vi "Wire All Terminals_core.vi"(8 "error in (no error)":errorcluster, 9 "User string":string, 10 "Create constants?":bool, 11 "SelList[]":refnum<vi>[](array[refnum])) -> (0 "error out":errorcluster, 3 "changes made?":bool)   [LabVIEW 2020]
doc: "Creates controls and indicators for all unwired inputs and outputs of the selected block diagram object(s). If 'shift' is also pressed, creates constants for all unwired inputs of the selected block diagram object(s).\n\nDefault Shortcut - [D]"
uses:
  <resource>/plugins/PopupMenus/edit time panel and diagram/zzRemove (no error).llb/zzRemove (no error).ctl
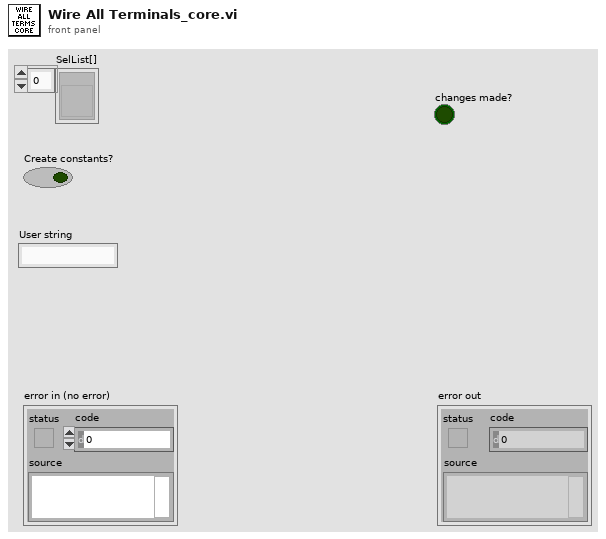
[diagram p1: front panel]
types:
  T1 = typedef "zzRemove (no error).ctl" = cluster{"Terminals":refnum<vi>[]}
  T2 = enum16{"Invalid Wire Rule", "Required", "Recommended", "Optional", "Dynamic Dispatch"}[]
  T3 = typedef "NI_Data Type.lvlib/Data Type.ctl" = enum8{"Invalid Type", "Void", "I8", "I16", "I32", "I64", "U8", "U16", "U32", "U64", "Single Float", "Double Float", "Extended Float", "Single Complex", "Double Complex", "Extended Complex", "Enum U8", "Enum U16", "Enum U32", "Enum U64", "Single Float With Unit", "Double Float With Unit", "Extended Float With Unit", "Single Complex with Unit", "Double Complex with Unit", "Extended Complex with Unit", "Boolean", "String", "Path", "Picture", "Tag", "Array", "Cluster", "Variant", "LV Variant", "Waveform", "Timestamp", "Digital Waveform", "Digital Data", "ExpressData", "Refnum", "External Data", "VI", "Poly VI", "LabVIEW Class Instance", "Fixed Point", "Set Collection", "Map Collection"}
  T4 = enum16{"Invalid Wire Rule", "Required", "Recommended", "Optional"}
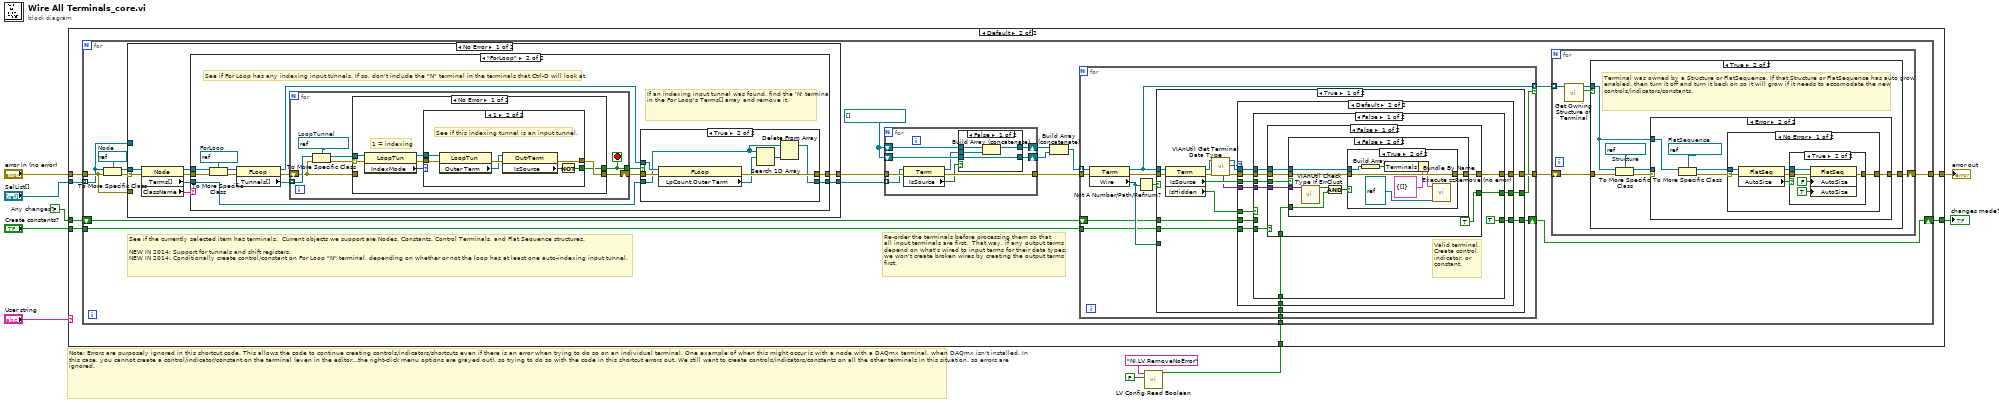
[diagram p0: block diagram]
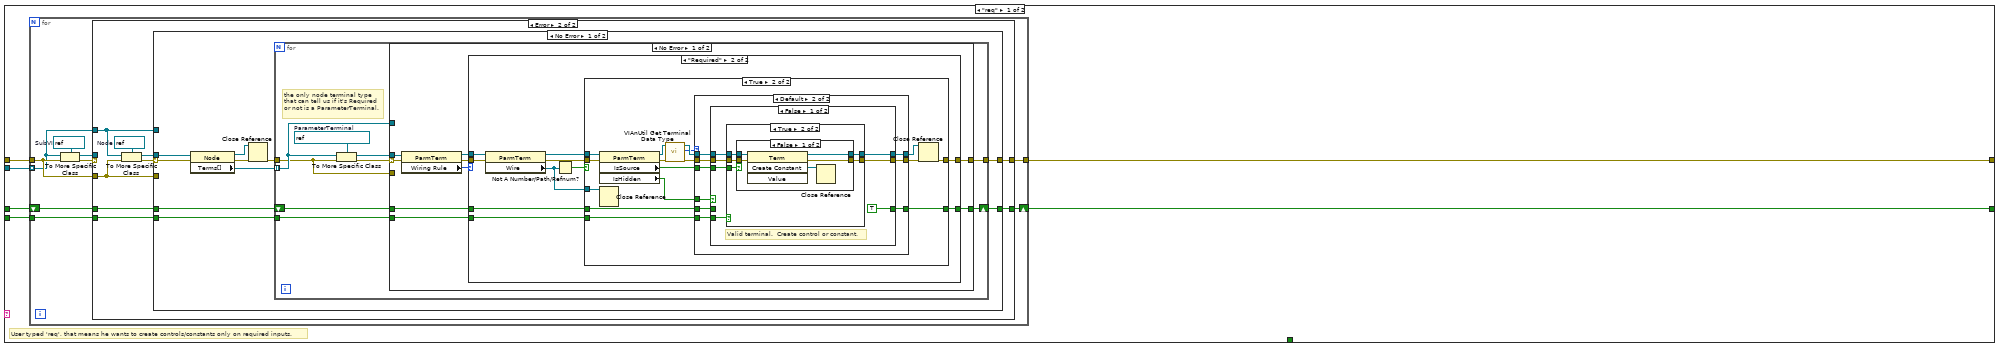
[diagram p2: hidden frame]
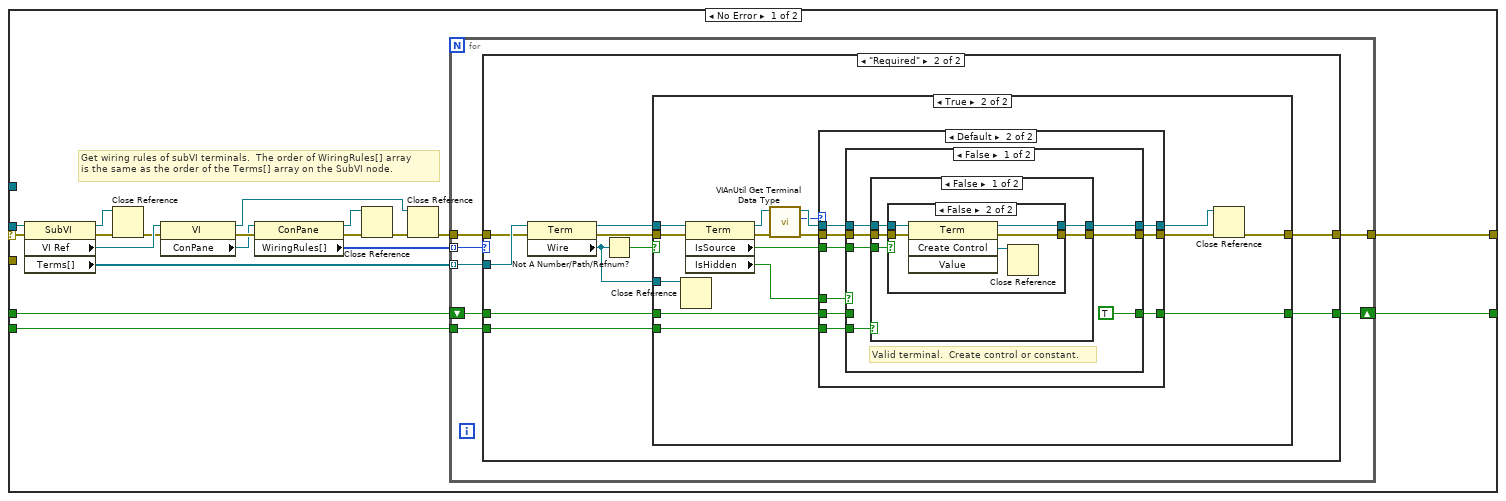
[diagram p3: hidden frame]
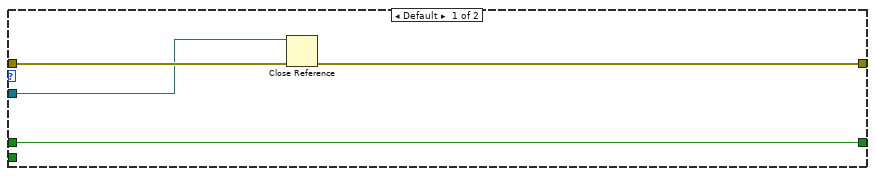
[diagram p4: hidden frame]
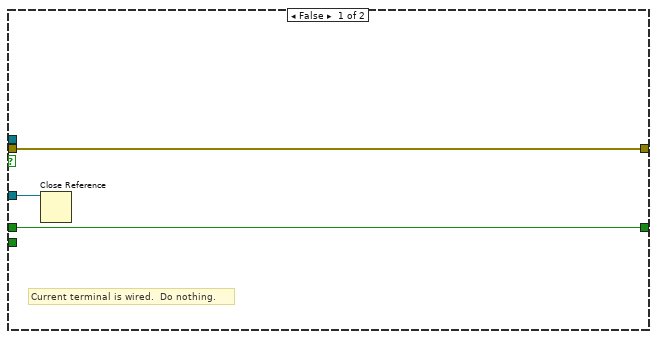
[diagram p5: hidden frame]
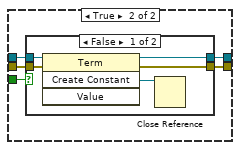
[diagram p8: hidden frame]
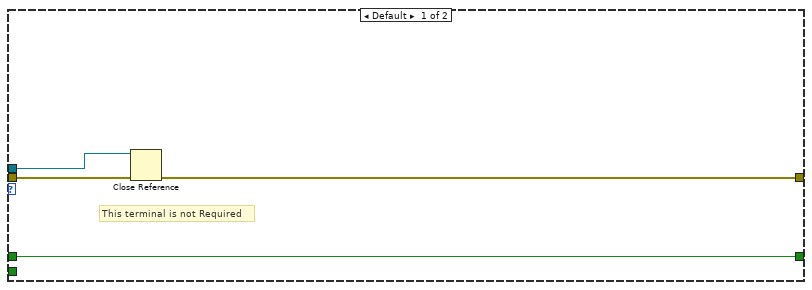
[diagram p11: hidden frame]
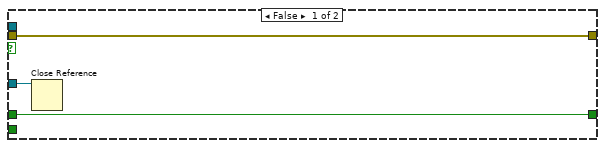
[diagram p12: hidden frame]
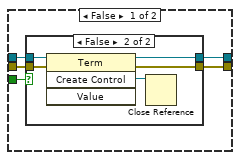
[diagram p14: hidden frame]
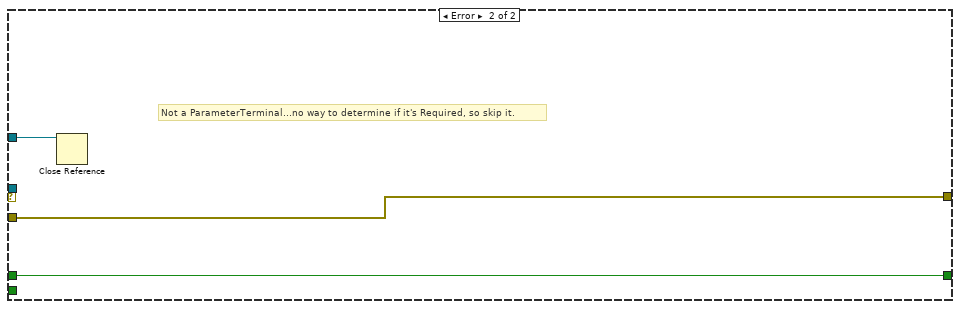
[diagram p18: hidden frame]
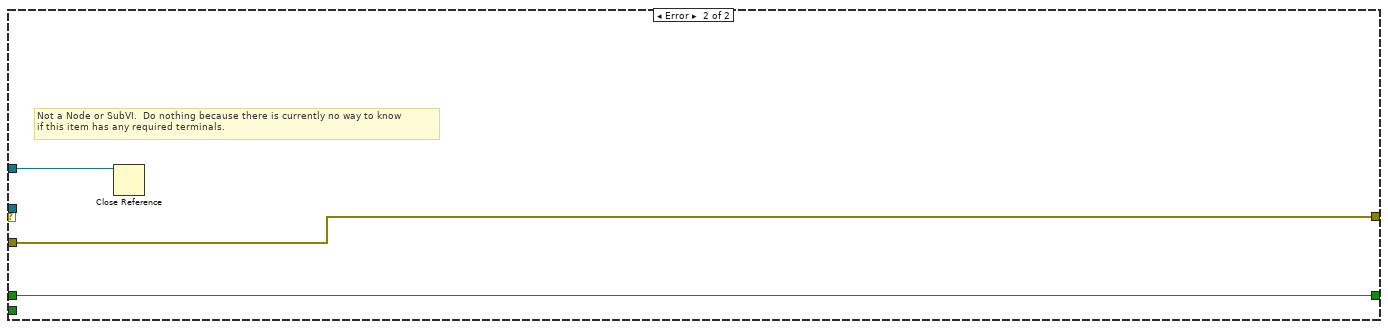
[diagram p19: hidden frame]
diagram:
  w10 = FALSE  # Any changes?
  # "Note: Errors are purposely ignored in this shortcut code. This allows the code to continue creating controls/indicators/shortcuts even if there is an error when trying to do so on an individual terminal. One example of when this might occur is with a node with a DAQmx terminal, when DAQmx isn't installed. In this case, you cannot create a control/indicator/constant on the terminal (even in the editor...the right-click menu options are grayed out), so trying to do so with the code in this shortcut errors out. We still want to create controls/indicators/constants on all the other terminals in this situation, so errors are ignored."
  n1 = call <resource>:"LV Config Read Boolean.vi"("default value"=FALSE, "key"="NI.LV.RemoveNoError") -> ("value"=w1:bool)  [unwired: 3 in, 2 out]
  n2 = case shown="Default" "User string" {
    tunnel: "Create constants?" -> [w11 w259]
    tunnel: w10 -> [w16 w258]
    tunnel: [w15 w257] -> w7
    tunnel: [w12 w256] -> w8
    tunnel: "SelList[]" -> [w14 w255]
    tunnel: "error in (no error)" -> [w13 w254]
    tunnel: w1 -> [_ w253]
    frame "req" {
      # "User typed 'req', that means he wants to create controls/constants only on required inputs."
      n3 = for {
        shift-right: [w20] -> w15
        shift-left: w16 -> [w22]
        tunnel: w14 -> [w17] mode=indexing
        tunnel: w11 -> [w19]
        tunnel: w13 -> [w18]
        tunnel: [w21] -> w12
        w25 = refnum<vi> refnum  # SubVI
        n4 = To More Specific Class(target class=w25, reference=w17, error in=w18) -> (specific class reference=w23:refnum<vi>, error out=w24:errorcluster)
        n5 = case shown="Error" w24 {
          selector: w24 -> [w43 _]
          tunnel: w23 -> [w44 _]
          tunnel: w22 -> [w30 w132]
          tunnel: [w33 w134] -> w21
          tunnel: [w29 w133] -> w20
          tunnel: w19 -> [w28 w131]
          tunnel: w18 -> [_ w137]
          tunnel: w17 -> [_ w135]
          frame No Error {
            # "Get wiring rules of subVI terminals.  The order of WiringRules[] array\nis the same as the order of the Terms[] array on the SubVI node."
            n6 = property class="SubVI"(reference=w44, error in=w43) -> (reference out=w26:refnum<vi>, error out=w42:errorcluster, "VI Ref"=w41:refnum<vi>, "Terms[]"=w31:refnum<vi>[])
            n7 = Close Reference(reference=w26, error in (no error)=w42) -> (error out=w27:errorcluster)
            n8 = property class="VI"(reference=w41, error in=w27) -> (reference out=w35:refnum<vi>, error out=w40:errorcluster, "ConPane"=w39:refnum<vi>)
            n9 = property class="ConPane"(reference=w39, error in=w40) -> (reference out=w37:refnum<vi>, error out=w38:errorcluster, "WiringRules[]"=w32:T2)
            n10 = Close Reference(reference=w37, error in (no error)=w38) -> (error out=w36:errorcluster)
            n11 = Close Reference(reference=w35, error in (no error)=w36) -> (error out=w34:errorcluster)
            n12 = for {
              tunnel: w32 -> [w50] mode=indexing
              tunnel: w31 -> [w49] mode=indexing
              shift-right: [w46] -> w29
              shift-left: w30 -> [w47]
              tunnel: w28 -> [w45]
              tunnel: w34 -> [w51]
              tunnel: [w48] -> w33
              n13 = case shown="\"Required\"" w50 {
                tunnel: w51 -> [w55 w57]
                tunnel: w49 -> [w52 w61]
                tunnel: [w54 w62] -> w48
                tunnel: w47 -> [w53 w65]
                tunnel: [w53 w63] -> w46
                tunnel: w45 -> [_ w64]
                frame Default {
                  n14 = Close Reference(reference=w52, error in (no error)=w55) -> (error out=w54:errorcluster)
                }
                frame "Required" {
                  n15 = property class="Term"(reference=w61, error in=w57) -> (reference out=w60:refnum<vi>, error out=w56:errorcluster, "Wire"=w58:refnum<vi>)
                  n16 = Not A Number/Path/Refnum?(number/path/refnum=w58) -> (NaN/Path/Refnum?=w59:bool)
                  n17 = case shown="True" w59 {
                    tunnel: w65 -> [w66 w80]
                    tunnel: w64 -> [_ w79]
                    tunnel: [w66 w78] -> w63
                    tunnel: [w67 w77] -> w62
                    tunnel: w56 -> [w67 w76]
                    tunnel: w60 -> [_ w70]
                    tunnel: w58 -> [w68 w69]
                    frame False {
                      # "Current terminal is wired.  Do nothing."
                      n18 = Close Reference(reference=w68) -> ()  [unwired: 1 in, 1 out]
                    }
                    frame True {
                      n19 = Close Reference(reference=w69) -> ()  [unwired: 1 in, 1 out]
                      n20 = property class="Term"(reference=w70, error in=w76) -> (reference out=w73:refnum<vi>, error out=w75:errorcluster, "IsSource"=w84:bool, "IsHidden"=w81:bool)
                      n21 = call <vilib>:"VIAnUtil Get Terminal Data Type.vi"("error in (no error)"=w75, "Terminal in"=w73) -> ("error out"=w74:errorcluster, "Data Type"=w71:T3, "Terminal out"=w72:refnum<vi>)  [unwired: 6 in, 1 out]
                      n22 = case shown="Default" w71 {
                        tunnel: [w87 w96] -> w78
                        tunnel: w84 -> [_ w95]
                        tunnel: w72 -> [w85 w94]
                        tunnel: [w86 w93] -> w83
                        tunnel: [w85 w92] -> w82
                        tunnel: w74 -> [w86 w91]
                        tunnel: w80 -> [w87 w88]
                        tunnel: w79 -> [_ w90]
                        tunnel: w81 -> [_ w89]
                        frame "Invalid Type", "Void" {
                          # "Current terminal is void (like an empty terminal on\na subVI).  Do nothing."
                        }
                        frame Default {
                          n23 = case shown="False" w89 {
                            tunnel: [TRUE w128] -> w96
                            tunnel: w95 -> [w102 _]
                            tunnel: w94 -> [w101 w129]
                            tunnel: [w100 w130] -> w93
                            tunnel: [w99 w129] -> w92
                            tunnel: w91 -> [w98 w130]
                            tunnel: w90 -> [w97 _]
                            tunnel: w88 -> [_ w128]
                            frame False {
                              # "Valid terminal.  Create control or constant."
                              n24 = case shown="False" w97 {
                                tunnel: w102 -> [w108 w120]
                                tunnel: w101 -> [w107 w119]
                                tunnel: [w106 w118] -> w100
                                tunnel: [w105 w117] -> w99
                                tunnel: w98 -> [w104 w116]
                                frame False {
                                n25 = case shown="False" w108 {
                                tunnel: w104 -> [w109 w115]
                                tunnel: w107 -> [w110 w113]
                                tunnel: [w109 w114] -> w106
                                tunnel: [w110 w112] -> w105
                                frame True {
                                }
                                frame False {
                                n26 = invoke class="Term" method="Create Control"(reference=w113, error in=w115) -> (reference out=w112:refnum<vi>, error out=w114:errorcluster, "Create Control"=w111:refnum<vi>)  [unwired: 2 in, 1 out]
                                n27 = Close Reference(reference=w111) -> ()  [unwired: 1 in, 1 out]
                                }
                                }
                                }
                                frame True {
                                n28 = case shown="False" w120 {
                                tunnel: w116 -> [w125 w127]
                                tunnel: w119 -> [w123 w126]
                                tunnel: [w124 w127] -> w118
                                tunnel: [w122 w126] -> w117
                                frame False {
                                n29 = invoke class="Term" method="Create Constant"(reference=w123, error in=w125) -> (reference out=w122:refnum<vi>, error out=w124:errorcluster, "Create Constant"=w121:refnum<vi>)  [unwired: 2 in, 1 out]
                                n30 = Close Reference(reference=w121) -> ()  [unwired: 1 in, 1 out]
                                }
                                frame True {
                                }
                                }
                                }
                              }
                            }
                            frame True {
                              # "Do not attempt to create inputs/outputs\non hidden terminals (like Dynamic Event terms\non an Event Structure that aren't showing)"
                            }
                          }
                        }
                      }
                      n31 = Close Reference(reference=w82, error in (no error)=w83) -> (error out=w77:errorcluster)
                    }
                  }
                }
              }
            }
          }
          frame Error {
            w139 = refnum<vi> refnum  # Node
            n32 = To More Specific Class(target class=w139, reference=w135, error in=w137) -> (specific class reference=w136:refnum<vi>, error out=w138:errorcluster)
            n33 = case shown="No Error" w138 {
              selector: w138 -> [w149 _]
              tunnel: w137 -> [_ w251]
              tunnel: w136 -> [w148 _]
              tunnel: w135 -> [_ w252]
              tunnel: [w141 w251] -> w134
              tunnel: [w142 w250] -> w133
              tunnel: w132 -> [w143 w250]
              tunnel: w131 -> [w140 _]
              frame No Error {
                n34 = property class="Node"(reference=w148, error in=w149) -> (reference out=w146:refnum<vi>, error out=w147:errorcluster, "Terms[]"=w144:refnum<vi>[])
                n35 = Close Reference(reference=w146, error in (no error)=w147) -> (error out=w145:errorcluster)
                n36 = for {
                  tunnel: w144 -> [w153] mode=indexing
                  shift-right: [w154] -> w142
                  shift-left: w143 -> [w155]
                  tunnel: w140 -> [w150]
                  tunnel: w145 -> [w152]
                  tunnel: [w151] -> w141
                  w158 = refnum<vi> refnum  # ParameterTerminal
                  # "the only node terminal type\nthat can tell us if it's Required\nor not is a ParameterTerminal."
                  n37 = To More Specific Class(target class=w158, reference=w153, error in=w152) -> (specific class reference=w156:refnum<vi>, error out=w157:errorcluster)
                  n38 = case shown="No Error" w157 {
                    selector: w157 -> [w167 _]
                    tunnel: w156 -> [w166 _]
                    tunnel: w155 -> [w165 w249]
                    tunnel: [w160 w249] -> w154
                    tunnel: w153 -> [_ w248]
                    tunnel: w152 -> [_ w247]
                    tunnel: [w161 w247] -> w151
                    tunnel: w150 -> [w159 _]
                    frame No Error {
                      n39 = property class="ParmTerm"(reference=w166, error in=w167) -> (reference out=w162:refnum<vi>, error out=w163:errorcluster, "Wiring Rule"=w164:T4)
                      n40 = case shown="\"Required\"" w164 {
                        tunnel: w165 -> [w168 w181]
                        tunnel: w163 -> [w171 w175]
                        tunnel: w162 -> [w170 w177]
                        tunnel: [w169 w179] -> w161
                        tunnel: [w168 w180] -> w160
                        tunnel: w159 -> [_ w178]
                        frame Default {
                          # "This terminal is not Required"
                          n41 = Close Reference(reference=w170, error in (no error)=w171) -> (error out=w169:errorcluster)
                        }
                        frame "Required" {
                          n42 = property class="ParmTerm"(reference=w177, error in=w175) -> (reference out=w176:refnum<vi>, error out=w174:errorcluster, "Wire"=w172:refnum<vi>)
                          n43 = Not A Number/Path/Refnum?(number/path/refnum=w172) -> (NaN/Path/Refnum?=w173:bool)
                          n44 = case shown="True" w173 {
                            tunnel: w176 -> [_ w196]
                            tunnel: w181 -> [w184 w195]
                            tunnel: [w184 w194] -> w180
                            tunnel: [w183 w193] -> w179
                            tunnel: w178 -> [_ w192]
                            tunnel: w174 -> [w183 w191]
                            tunnel: w172 -> [w182 w185]
                            frame False {
                              n45 = Close Reference(reference=w182) -> ()  [unwired: 1 in, 1 out]
                            }
                            frame True {
                              n46 = property class="ParmTerm"(reference=w196, error in=w191) -> (reference out=w189:refnum<vi>, error out=w190:errorcluster, "IsSource"=w200:bool, "IsHidden"=w197:bool)
                              n47 = Close Reference(reference=w185) -> ()  [unwired: 1 in, 1 out]
                              n48 = call <vilib>:"VIAnUtil Get Terminal Data Type.vi"("error in (no error)"=w190, "Terminal in"=w189) -> ("error out"=w187:errorcluster, "Data Type"=w186:T3, "Terminal out"=w188:refnum<vi>)  [unwired: 6 in, 1 out]
                              n49 = case shown="Default" w186 {
                                tunnel: [w203 w212] -> w194
                                tunnel: w200 -> [_ w211]
                                tunnel: w188 -> [w201 w210]
                                tunnel: [w202 w209] -> w199
                                tunnel: [w201 w208] -> w198
                                tunnel: w187 -> [w202 w207]
                                tunnel: w195 -> [w203 w204]
                                tunnel: w192 -> [_ w206]
                                tunnel: w197 -> [_ w205]
                                frame "Invalid Type", "Void" {
                                # "Current terminal is void (like an empty terminal on\na subVI).  Do nothing."
                                }
                                frame Default {
                                n50 = case shown="False" w205 {
                                tunnel: [TRUE w244] -> w212
                                tunnel: w211 -> [w218 _]
                                tunnel: w210 -> [w217 w245]
                                tunnel: [w216 w246] -> w209
                                tunnel: [w215 w245] -> w208
                                tunnel: w207 -> [w214 w246]
                                tunnel: w206 -> [w213 _]
                                tunnel: w204 -> [_ w244]
                                frame False {
                                # "Valid terminal.  Create control or constant."
                                n51 = case shown="True" w213 {
                                tunnel: w218 -> [w224 w236]
                                tunnel: w217 -> [w223 w235]
                                tunnel: [w222 w234] -> w216
                                tunnel: [w221 w233] -> w215
                                tunnel: w214 -> [w220 w232]
                                frame False {
                                n52 = case shown="False" w224 {
                                tunnel: w220 -> [w225 w231]
                                tunnel: w223 -> [w226 w229]
                                tunnel: [w225 w230] -> w222
                                tunnel: [w226 w228] -> w221
                                frame True {
                                }
                                frame False {
                                n53 = invoke class="Term" method="Create Control"(reference=w229, error in=w231) -> (reference out=w228:refnum<vi>, error out=w230:errorcluster, "Create Control"=w227:refnum<vi>)  [unwired: 2 in, 1 out]
                                n54 = Close Reference(reference=w227) -> ()  [unwired: 1 in, 1 out]
                                }
                                }
                                }
                                frame True {
                                n55 = case shown="False" w236 {
                                tunnel: w232 -> [w241 w243]
                                tunnel: w235 -> [w239 w242]
                                tunnel: [w240 w243] -> w234
                                tunnel: [w238 w242] -> w233
                                frame False {
                                n56 = invoke class="Term" method="Create Constant"(reference=w239, error in=w241) -> (reference out=w238:refnum<vi>, error out=w240:errorcluster, "Create Constant"=w237:refnum<vi>)  [unwired: 2 in, 1 out]
                                n57 = Close Reference(reference=w237) -> ()  [unwired: 1 in, 1 out]
                                }
                                frame True {
                                }
                                }
                                }
                                }
                                }
                                frame True {
                                # "Do not attempt to create inputs/outputs\non hidden terminals (like Dynamic Event terms\non an Event Structure that aren't showing)"
                                }
                                }
                                }
                              }
                              n58 = Close Reference(reference=w198, error in (no error)=w199) -> (error out=w193:errorcluster)
                            }
                          }
                        }
                      }
                    }
                    frame Error {
                      # "Not a ParameterTerminal...no way to determine if it's Required, so skip it."
                      n59 = Close Reference(reference=w248) -> ()  [unwired: 1 in, 1 out]
                    }
                  }
                }
              }
              frame Error {
                # "Not a Node or SubVI.  Do nothing because there is currently no way to know\nif this item has any required terminals."
                n60 = Close Reference(reference=w252) -> ()  [unwired: 1 in, 1 out]
              }
            }
          }
        }
      }
    }
    frame Default {
      n61 = for {
        tunnel: w255 -> [w272] mode=indexing
        shift-right: [w261] -> w257
        shift-left: w258 -> [w276]
        tunnel: w259 -> [w275]
        tunnel: w254 -> [w274]
        tunnel: [w263] -> w256
        tunnel: w253 -> [w260]
        w267 = refnum<vi>[] [] ("Terms[]")
        w278 = refnum<vi> refnum  # Node
        # "Re-order the terminals before processing them so that\nall input terminals are first.  That way, if any output terms\ndepend on what's wired to input terms for their data types,\nwe won't create broken wires by creating the output terms\nfirst."
        # "See if the currently selected item has terminals.  Current objects we support are Nodes, Constants, Control Terminals, and Flat Sequence structures.\n\nNEW IN 2014: Support for tunnels and shift registers.\nNEW IN 2014: Conditionally create control/constant on For Loop \"N\" terminal, depending on whether or not the loop has at least one auto-indexing input tunnel."
        n62 = To More Specific Class(target class=w278, reference=w272, error in=w274) -> (specific class reference=w277:refnum<vi>, error out=w273:errorcluster)
        n63 = case shown="No Error" w273 {
          selector: w273 -> [w343 _]
          tunnel: w277 -> [w344 _]
          tunnel: [w338 w393] -> w270
          tunnel: [w339 w394] -> w271
          tunnel: w274 -> [_ w395]
          tunnel: w272 -> [_ w392]
          frame No Error {
            n64 = property class="Node"(reference=w344, error in=w343) -> (reference out=w337:refnum<vi>, error out=w340:errorcluster, "Terms[]"=w341:refnum<vi>[], "ClassName"=w342:string)
            n65 = case shown="\"ForLoop\"" w342 {
              tunnel: w341 -> [w345 w350]
              tunnel: w340 -> [w346 w359]
              tunnel: [w346 w348] -> w339
              tunnel: [w345 w349] -> w338
              tunnel: w337 -> [_ w358]
              frame Default {
                # "Node is not a For Loop."
              }
              frame "ForLoop" {
                w357 = refnum<vi> refnum  # ForLoop
                # "If an indexing input tunnel was found, find the 'N' terminal in the For Loop's Terms[] array and remove it."
                # "See if For Loop has any indexing input tunnels. If so, don't include the \"N\" terminal in the terminals that Ctrl-D will look at."
                n66 = To More Specific Class(target class=w357, reference=w358, error in=w359) -> (specific class reference=w355:refnum<vi>, error out=w356:errorcluster)
                n67 = property class="FLoop"(reference=w355, error in=w356) -> (reference out=w347:refnum<vi>, error out=w354:errorcluster, "Tunnels[]"=w353:refnum<vi>[])
                n68 = for {
                  shift-right: [w370] -> w352
                  shift-left: w354 -> [w373]
                  tunnel: w353 -> [w374] mode=indexing
                  tunnel: [w369] -> w351
                  stop <- w369 stop-if-true
                  w375 = refnum<vi> refnum  # LoopTunnel
                  n69 = To More Specific Class(target class=w375, reference=w374, error in=w373) -> (specific class reference=w371:refnum<vi>, error out=w372:errorcluster)
                  n70 = case shown="No Error" w372 {
                    selector: w372 -> [w382 _]
                    tunnel: w373 -> [_ w391]
                    tunnel: w371 -> [w381 _]
                    tunnel: [w377 w391] -> w370
                    tunnel: [w376 _] -> w369
                    frame No Error {
                      # "1 = indexing"
                      n71 = property class="LoopTun"(reference=w381, error in=w382) -> (reference out=w378:refnum<vi>, error out=w379:errorcluster, "IndexMode"=w380:u32)
                      n72 = case shown="1" w380 {
                        tunnel: w379 -> [w383 w390]
                        tunnel: w378 -> [_ w389]
                        tunnel: [w383 w386] -> w377
                        tunnel: [_ w384] -> w376
                        frame Default {
                          # "Not an indexing loop tunnel"
                        }
                        frame 1 {
                          # "See if this indexing tunnel is an input tunnel."
                          n73 = property class="LoopTun"(reference=w389, error in=w390) -> (error out=w388:errorcluster, "Outer Term"=w387:refnum<vi>)  [unwired: 1 out]
                          n74 = property class="OutrTerm"(reference=w387, error in=w388) -> (error out=w386:errorcluster, "IsSource"=w385:bool)  [unwired: 1 out]
                          n75 = Not(x=w385) -> (.not. x?=w384:bool)
                        }
                      }
                    }
                    frame Error {
                      # "Not a LoopTunnel, so indexing can't be set on it."
                    }
                  }
                }
                n76 = case shown="True" w351 {
                  tunnel: w352 -> [w360 w368]
                  tunnel: w350 -> [w361 w363]
                  tunnel: [w361 w362] -> w349
                  tunnel: [w360 w366] -> w348
                  tunnel: w347 -> [_ w367]
                  frame False {
                  }
                  frame True {
                    n77 = property class="FLoop"(reference=w367, error in=w368) -> (error out=w366:errorcluster, "LpCount.Outer Term"=w365:refnum<vi>)  [unwired: 1 out]
                    n78 = Search 1D Array(1D array=w363, element=w365) -> (index of element=w364:i32)  [unwired: 1 in]
                    n79 = Delete From Array(array=w363, index=w364) -> (array with subset deleted=w362:refnum<vi>[])  [unwired: 1 in, 1 out]
                  }
                }
              }
            }
          }
          frame Error {
            w398 = refnum<vi> refnum  # Constant
            n80 = To More Specific Class(target class=w398, reference=w392, error in=w395) -> (specific class reference=w396:refnum<vi>, error out=w397:errorcluster)
            n81 = case shown="Error" w397 {
              selector: w397 -> [w405 _]
              tunnel: w395 -> [_ w407]
              tunnel: w396 -> [w404 _]
              tunnel: [w399 w409] -> w394
              tunnel: [w402 w408] -> w393
              tunnel: w392 -> [_ w406]
              frame No Error {
                n82 = property class="Const"(reference=w404, error in=w405) -> (reference out=w400:refnum<vi>, error out=w401:errorcluster, "Terminal"=w403:refnum<vi>)
                n83 = Close Reference(reference=w400, error in (no error)=w401) -> (error out=w399:errorcluster)
                n84 = Build Array(w403) -> (w402:refnum<vi>[])
              }
              frame Error {
                w412 = refnum<vi> refnum  # Terminal
                n85 = To More Specific Class(target class=w412, reference=w406, error in=w407) -> (specific class reference=w410:refnum<vi>, error out=w411:errorcluster)
                n86 = case shown="Error" w411 {
                  selector: w411 -> [w415 _]
                  tunnel: w410 -> [w414 _]
                  tunnel: [w415 w418] -> w409
                  tunnel: [w413 w417] -> w408
                  tunnel: w407 -> [_ w419]
                  tunnel: w406 -> [_ w416]
                  frame No Error {
                    n87 = Build Array(w414) -> (w413:refnum<vi>[])
                  }
                  frame Error {
                    w422 = refnum<vi> refnum  # FlatSequence
                    n88 = To More Specific Class(target class=w422, reference=w416, error in=w419) -> (specific class reference=w420:refnum<vi>, error out=w421:errorcluster)
                    n89 = case shown="Error" w421 {
                      selector: w421 -> [w428 _]
                      tunnel: w420 -> [w427 _]
                      tunnel: w419 -> [_ w431]
                      tunnel: [w423 w430] -> w418
                      tunnel: [w426 w429] -> w417
                      tunnel: w416 -> [_ w432]
                      frame No Error {
                        n90 = property class="FlatSeq"(reference=w427, error in=w428) -> (reference out=w424:refnum<vi>, error out=w425:errorcluster, "Terms[]"=w426:refnum<vi>[])
                        n91 = Close Reference(reference=w424, error in (no error)=w425) -> (error out=w423:errorcluster)
                      }
                      frame Error {
                        w435 = refnum<vi> refnum  # Tunnel
                        n92 = To More Specific Class(target class=w435, reference=w432, error in=w431) -> (specific class reference=w433:refnum<vi>, error out=w434:errorcluster)
                        n93 = case shown="No Error" w434 {
                          selector: w434 -> [w440 _]
                          tunnel: w433 -> [w439 _]
                          tunnel: w432 -> [_ _]
                          tunnel: w431 -> [_ w441]
                          tunnel: [w438 w441] -> w430
                          tunnel: [w436 _] -> w429
                          frame No Error {
                            # "Get the outside terminal of any selected tunnel. This also includes shift registers (they inherit from the Tunnel class)."
                            n94 = property class="Tun"(reference=w439, error in=w440) -> (error out=w438:errorcluster, "Outer Term"=w437:refnum<vi>)  [unwired: 1 out]
                            n95 = Build Array(w437) -> (w436:refnum<vi>[])
                          }
                          frame Error {
                            # "Not a supported type for this shortcut."
                          }
                        }
                      }
                    }
                  }
                }
              }
            }
          }
        }
        n96 = for {
          tunnel: w270 -> [w327] mode=indexing
          shift-right: [w323] -> w266
          shift-left: w267 -> [w325]
          shift-right: [w322] -> w265
          shift-left: w267 -> [w324]
          tunnel: w271 -> [w328]
          tunnel: [w326] -> w269
          n97 = property class="Term"(reference=w327, error in=w328) -> (reference out=w321:refnum<vi>, error out=w326:errorcluster, "IsSource"=w320:bool)
          n98 = case shown="False" w320 {
            tunnel: w325 -> [w332 w336]
            tunnel: w324 -> [w330 w335]
            tunnel: [w331 w336] -> w323
            tunnel: [w330 w334] -> w322
            tunnel: w321 -> [w329 w333]
            frame False {
              n99 = Build Array (concatenate)(w332, w329) -> (w331:refnum<vi>[])
            }
            frame True {
              n100 = Build Array (concatenate)(w335, w333) -> (w334:refnum<vi>[])
            }
          }
        }
        n101 = Build Array (concatenate)(w266, w265) -> (w268:refnum<vi>[])
        n102 = for {
          tunnel: w268 -> [w452] mode=indexing
          shift-right: [w447] -> w261
          shift-left: w276 -> [w448]
          tunnel: w275 -> [w445]
          tunnel: w269 -> [w453]
          tunnel: [w446] -> w264
          tunnel: [w444] -> w262 mode=indexing if=w443
          tunnel: w260 -> [w442]
          n103 = property class="Term"(reference=w452, error in=w453) -> (reference out=w444:refnum<vi>, error out=w451:errorcluster, "Wire"=w449:refnum<vi>)
          n104 = Not A Number/Path/Refnum?(number/path/refnum=w449) -> (NaN/Path/Refnum?=w450:bool)
          n105 = case shown="True" w450 {
            tunnel: w451 -> [w469 w530]
            tunnel: w444 -> [w468 _]
            tunnel: w449 -> [_ _]
            tunnel: w448 -> [w465 w531]
            tunnel: [w467 w531] -> w447
            tunnel: [w457 w530] -> w446
            tunnel: w445 -> [w464 _]
            tunnel: [w456 _] -> w443
            tunnel: w442 -> [w455 _]
            frame True {
              n106 = property class="Term"(reference=w468, error in=w469) -> (reference out=w460:refnum<vi>, error out=w462:errorcluster, "IsSource"=w466:bool, "IsHidden"=w463:bool)
              n107 = call <vilib>:"VIAnUtil Get Terminal Data Type.vi"("error in (no error)"=w462, "Terminal in"=w460) -> ("error out"=w461:errorcluster, "Data Type"=w458:T3, "Terminal out"=w459:refnum<vi>, "Type Variant"=w454:variant)  [unwired: 6 in]
              n108 = case shown="Default" w458 {
                tunnel: [w471 w482] -> w467
                tunnel: w466 -> [_ w481]
                tunnel: w459 -> [_ w480]
                tunnel: [w470 w479] -> w457
                tunnel: w461 -> [w470 w478]
                tunnel: w465 -> [w471 w475]
                tunnel: w464 -> [_ w477]
                tunnel: w463 -> [_ w476]
                tunnel: [_ w474] -> w456
                tunnel: w455 -> [_ w473]
                tunnel: w454 -> [_ w472]
                frame "Invalid Type", "Void" {
                  # "Current terminal is void (like an empty terminal on a subVI).  Do nothing."
                }
                frame Default {
                  n109 = case shown="False" w476 {
                    tunnel: [TRUE w528] -> w482
                    tunnel: w481 -> [w490 _]
                    tunnel: w480 -> [w489 _]
                    tunnel: [w488 w529] -> w479
                    tunnel: w478 -> [w487 w529]
                    tunnel: w477 -> [w486 _]
                    tunnel: w475 -> [_ w528]
                    tunnel: [w485 _] -> w474
                    tunnel: w473 -> [w484 _]
                    tunnel: w472 -> [w483 _]
                    frame False {
                      # "Valid terminal.  Create control, indicator, or constant."
                      n110 = case shown="False" w486 {
                        tunnel: w490 -> [w498 w522]
                        tunnel: w489 -> [w497 w521]
                        tunnel: [w496 w520] -> w488
                        tunnel: w487 -> [w495 w519]
                        tunnel: [TRUE w518] -> w485
                        tunnel: w484 -> [w493 _]
                        tunnel: w483 -> [w492 _]
                        frame False {
                          n111 = case shown="False" w498 {
                            tunnel: w495 -> [w501 w508]
                            tunnel: w497 -> [w499 w506]
                            tunnel: [w500 w507] -> w496
                            tunnel: w493 -> [_ w503]
                            tunnel: w492 -> [_ w505]
                            frame True {
                              n112 = invoke class="Term" method="Create Indicator"(reference=w499, error in=w501) -> (error out=w500:errorcluster)  [unwired: 1 in, 2 out]
                            }
                            frame False {
                              n113 = call <vilib>:"VIAnUtil Check Type If ErrClust.vi"("Data In"=w505) -> ("IsErrClust?"=w504:bool)  [unwired: 9 in, 1 out]
                              n114 = And(x=w504, y=w503) -> (x .and. y?=w502:bool)
                              n115 = case shown="True" w502 {
                                tunnel: w508 -> [w511 w517]
                                tunnel: [w510 w517] -> w507
                                tunnel: w506 -> [w509 w513]
                                frame False {
                                n116 = invoke class="Term" method="Create Control"(reference=w509, error in=w511) -> (error out=w510:errorcluster)  [unwired: 2 in, 3 out]
                                }
                                frame True {
                                n117 = Build Array(w513) -> (w514:refnum<vi>[])
                                n118 = Bundle By Name(cluster=T1 {"Terminals"=[]} ("Affected Items"), "Terminals"=w514) -> (w515:T1)
                                n119 = call <resource>:"Execute zzRemove (no error).vi"("User VI Ref"=refnum<vi> refnum, "Affected Items"=w515) -> ()  [unwired: 9 in, 1 out]
                                }
                              }
                            }
                          }
                        }
                        frame True {
                          n120 = case shown="False" w522 {
                            tunnel: w519 -> [w526 w527]
                            tunnel: w521 -> [w524 _]
                            tunnel: [w525 w527] -> w520
                            tunnel: [TRUE _] -> w518
                            frame False {
                              n121 = invoke class="Term" method="Create Constant"(reference=w524, error in=w526) -> (error out=w525:errorcluster)  [unwired: 2 in, 3 out]
                            }
                            frame True {
                            }
                          }
                        }
                      }
                    }
                    frame True {
                      # "Do not attempt to create inputs/outputs on hidden terminals (like Dynamic Event terms on an Event Structure that aren't showing)"
                    }
                  }
                }
              }
            }
            frame False {
              # "Current terminal is wired.  Do nothing."
            }
          }
        }
        n122 = for {
          shift-right: [w279] -> w263
          shift-left: w264 -> [w280]
          tunnel: w262 -> [w283] mode=indexing
          n123 = call <vilib>:"Get Owning Structure of Terminal.vi"("Terminal"=w283) -> ("Terminal Owned by Structure?"=w282:bool, "Owning Structure"=w281:refnum<vi>)  [unwired: 9 in]
          n124 = case shown="True" w282 {
            tunnel: w281 -> [_ w285]
            tunnel: w280 -> [w284 w290]
            tunnel: [w284 w286] -> w279
            frame False {
              # "Terminal was not owned at any point in its hierarchy by a Structure or FlatSequence. This terminal must be on the top-level diagram (or its owning Node is on the top-level diagram)."
            }
            frame True {
              w287 = refnum<vi> refnum  # Structure
              # "Terminal was owned by a Structure or FlatSequence. If that Structure or FlatSequence has auto grow enabled, then turn it off and turn it back on so it will grow if it needs to accomodate the new controls/indicators/constants."
              n125 = To More Specific Class(target class=w287, reference=w285, error in=w290) -> (specific class reference=w288:refnum<vi>, error out=w289:errorcluster)
              n126 = case shown="Error" w289 {
                selector: w289 -> [w296 _]
                tunnel: w288 -> [w295 _]
                tunnel: [w292 w303] -> w286
                tunnel: w285 -> [_ w306]
                frame No Error {
                  n127 = property class="Struct"(reference=w295, error in=w296) -> (reference out=w291:refnum<vi>, error out=w293:errorcluster, "AutoSize"=w294:bool)
                  n128 = case shown="True" w294 {
                    tunnel: w293 -> [w297 w301]
                    tunnel: [w297 w300] -> w292
                    tunnel: w291 -> [_ w302]
                    frame False {
                    }
                    frame True {
                      n129 = property class="Struct"(reference=w302, error in=w301, "AutoSize"=FALSE ("AutoSize To Fit Contents?"), "AutoSize"=TRUE ("AutoSize To Fit Contents?")) -> (error out=w300:errorcluster)  [unwired: 1 out]
                    }
                  }
                }
                frame Error {
                  w307 = refnum<vi> refnum  # FlatSequence
                  n130 = To More Specific Class(target class=w307, reference=w306) -> (specific class reference=w304:refnum<vi>, error out=w305:errorcluster)  [unwired: 1 in]
                  n131 = case shown="No Error" w305 {
                    selector: w305 -> [w310 _]
                    tunnel: w304 -> [w309 _]
                    tunnel: [w308 _] -> w303
                    frame No Error {
                      n132 = property class="FlatSeq"(reference=w309, error in=w310) -> (reference out=w311:refnum<vi>, error out=w312:errorcluster, "AutoSize"=w313:bool)
                      n133 = case shown="True" w313 {
                        tunnel: w312 -> [w314 w318]
                        tunnel: [w314 w317] -> w308
                        tunnel: w311 -> [_ w319]
                        frame False {
                        }
                        frame True {
                          n134 = property class="FlatSeq"(reference=w319, error in=w318, "AutoSize"=FALSE ("AutoSize To Fit Contents?"), "AutoSize"=TRUE ("AutoSize To Fit Contents?")) -> (error out=w317:errorcluster)  [unwired: 1 out]
                        }
                      }
                    }
                    frame Error {
                    }
                  }
                }
              }
            }
          }
        }
      }
    }
  }
  "error out" <- w8
  "changes made?" <- w7
